vi "Zero-Phase FIR Filter.vi"(3 "FIR Windowed Coefficients":dbl[](array[numeric]), 5 "Array":dbl[](array[numeric])) -> (2 "Filtered Array":dbl[](array[numeric]))   [LabVIEW 2020]
uses:
  <vilib>/Analysis/3filter.llb/FIR Filter (DBL).vi
  <vilib>/Analysis/NI_AALBase.lvlib
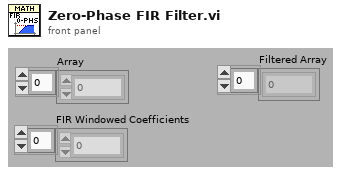
[diagram p1: front panel]
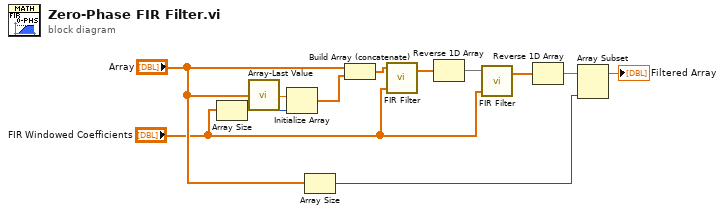
[diagram p0: block diagram]
diagram:
  n1 = Array Size(array="FIR Windowed Coefficients") -> (size(s)=w4:i32)
  n2 = call "Array-Last Value.vi"("array"="Array") -> ("element"=w7:dbl)
  n3 = Initialize Array(w7, w4) -> (w8:dbl[])
  n4 = Array Size(array="Array") -> (size(s)=w12:i32)
  n5 = Build Array (concatenate)("Array", w8) -> (w9:dbl[])
  n6 = call-poly <vilib>:"FIR Filter.vi"("FIR Coefficients"="FIR Windowed Coefficients", "X"=w9) -> ("Filtered X"=w5:dbl[])  [unwired: 2 in, 1 out]
  n7 = Reverse 1D Array(array=w5) -> (reversed array=w6:dbl[])
  n8 = call-poly <vilib>:"FIR Filter.vi"("FIR Coefficients"="FIR Windowed Coefficients", "X"=w6) -> ("Filtered X"=w3:dbl[])  [unwired: 2 in, 1 out]
  n9 = Reverse 1D Array(array=w3) -> (reversed array=w1:dbl[])
  n10 = Array Subset(array=w1, length=w12) -> (→"Filtered Array":dbl[])  [unwired: 1 in]
